vi "Get All Nodes of Names.vi"(8 "error in (no error)":errorcluster, 10 "Node Names":string[](array[string]), 11 "Project XML Editor in":refnum<class "Project XML Editor.lvclass">) -> (0 "error out":errorcluster, 2 "Nodes Array out":refnum<k20>[](array[refnum]), 3 "Project XML Editor out":refnum<class "Project XML Editor.lvclass">)   [LabVIEW 2018, in ".LVLIBP CD XML Updater.lvlib" / "Project XML Editor.lvclass"]
uses:
  Project XML Editor.lvclass
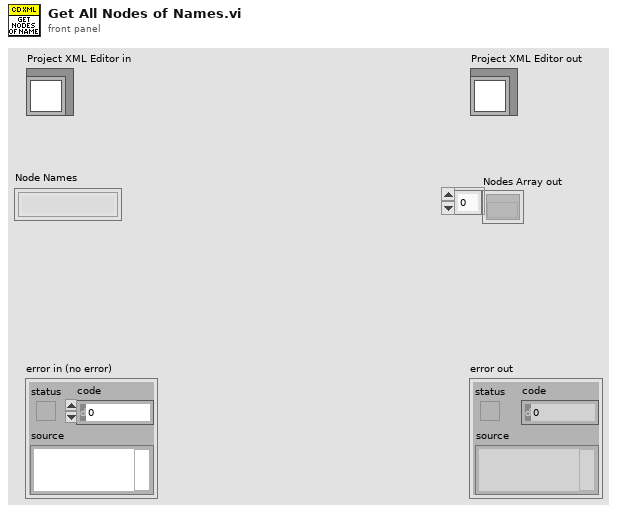
[diagram p1: front panel]
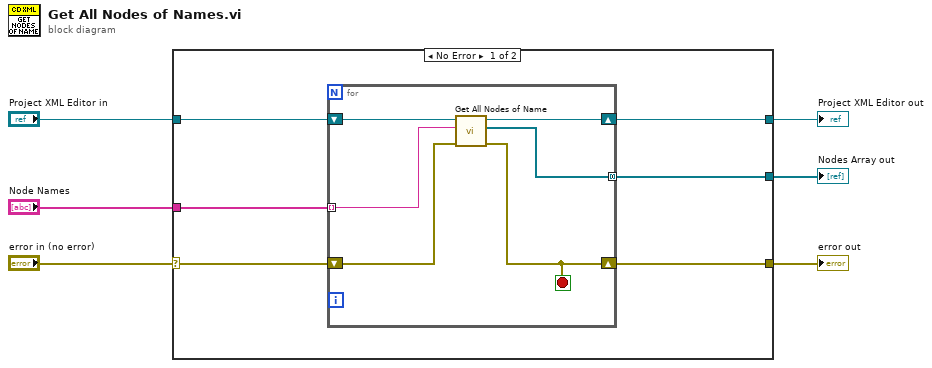
[diagram p0: block diagram]
diagram:
  n1 = case shown="No Error" "error in (no error)" {
    selector: "error in (no error)" -> [w10 w20]
    tunnel: [w7 w20] -> w5
    tunnel: [w8 w19] -> w3
    tunnel: "Project XML Editor in" -> [w11 w19]
    tunnel: "Node Names" -> [w12 _]
    tunnel: [w9 _] -> w1
    frame No Error {
      n2 = for {
        tunnel: w12 -> [w18] mode=indexing
        shift-right: [w16] -> w8
        shift-left: w11 -> [w17]
        tunnel: [w15] -> w9 mode=concatenating
        shift-right: [w13] -> w7
        shift-left: w10 -> [w14]
        stop <- w13 stop-if-true
        n3 = call "Get All Nodes of Name.vi"("error in (no error)"=w14, "Node Name"=w18, "Project XML Editor in"=w17) -> ("error out"=w13:errorcluster, "Nodes Array out"=w15:refnum<k20>[], "Project XML Editor out"=w16:refnum<class "Project XML Editor.lvclass">)  [unwired: 6 in]
      }
    }
    frame Error {
    }
  }
  "error out" <- w5
  "Project XML Editor out" <- w3
  "Nodes Array out" <- w1
